vi "getChamber.vi"(8 "error in (no error)":errorcluster, 11 "Instrument.Cryostat in":refnum<class "Instrument.Cryostat.lvclass">) -> (0 "error out":errorcluster, 2 "Status":string, 3 "Instrument.Cryostat out":refnum<class "Instrument.Cryostat.lvclass">)   [LabVIEW 2019, in "Instrument.Cryostat.lvclass"]
uses:
  Instrument.Cryostat.lvclass
  C:/Users/patrick/Documents/GitHub/Instrument-Framework/lvsrc/Framework/Instrument/Instrument.lvclass
  Typedefs/Cryostat.commands--enum.ctl
  adedcb00-9a43-4da2-8686-d28cc59b86bc.vi
  adedcb00-9a43-4da2-8686-d28cc59b86bc.vi/947f2777-6a3a-43f8-9da3-5ed9212fe224.vi
  adedcb00-9a43-4da2-8686-d28cc59b86bc.vi/2a6892e8-653d-450a-a90f-06ced07d9bc6.vi
  <vilib>/Utility/Data Type/Get Type Information.vi
  <vilib>/JDP Science/JSONtext/JSON text to Variant.vi
  <vilib>/JDP Science/JSONtext/LVClass Serializer/JSONtext LVClass Serializer.lvclass
  Instrument/Instrument.lvclass
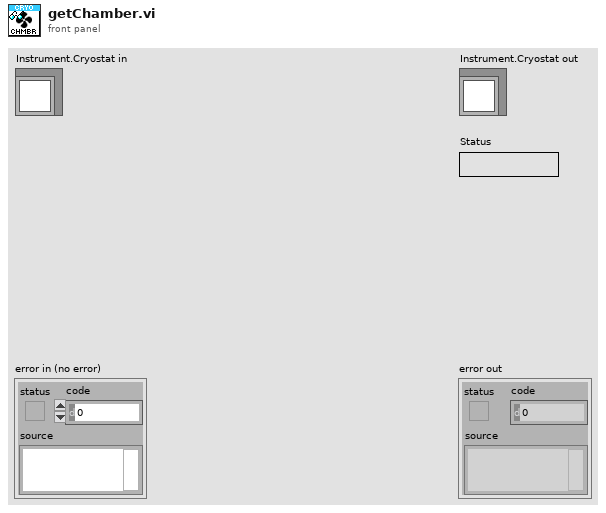
[diagram p1: front panel]
types:
  T1 = typedef "Instrument.Cryostat.lvclass/Cryostat.commands--enum.ctl" = enum16{"getLN2Level", "getLHeLevel", "getMagnet", "getMagnetVector", "setMagnet", "setMagnetVector", "getAngle", "setAngle", "getTemperature", "setTemperature", "getHeater", "setHeater", "getChamber", "setChamber", "getPressure"}
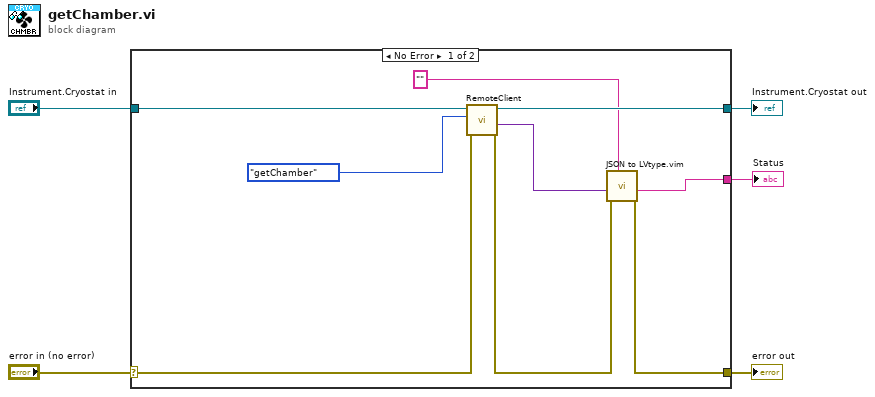
[diagram p0: block diagram]
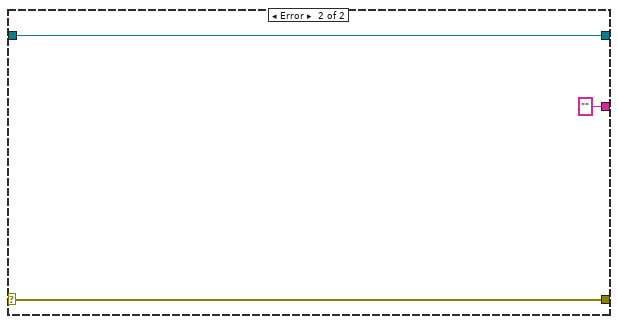
[diagram p2: hidden frame]
diagram:
  n1 = case shown="No Error" "error in (no error)" {
    selector: "error in (no error)" -> [w11 w17]
    tunnel: [w7 w17] -> w4
    tunnel: [w14 w16] -> w2
    tunnel: "Instrument.Cryostat in" -> [w12 w16]
    tunnel: [w6 "" ("Data out")] -> w1
    frame No Error {
      n2 = call "RemoteClient.vi"("error in (no error)"=w11, "Command in"=Cryostat.commands--enum."getChamber" ("commands"), "Instrument in"=w12) -> ("error out"=w8:errorcluster, "Data out"=w9:variant, "Instrument out"=w14:refnum<class "Instrument.Cryostat.lvclass">)  [unwired: 5 in, 1 out]
      n3 = call "JSON to LVtype.vim"("type"="", "error in (no error)"=w8, "JSON Data in"=w9) -> ("error out"=w7:errorcluster, "Data out"=w6:string)  [unwired: 7 in]
    }
    frame Error {
    }
  }
  "error out" <- w4
  "Instrument.Cryostat out" <- w2
  "Status" <- w1
